vi "Look right.vi"(8 "column":i32, 9 "row":i32, 10 "Tree":T1, 11 "Array":T1[][](array[typedef])) -> (2 "output cluster":T1)   [LabVIEW 2020]
uses:
  tree--cluster.ctl
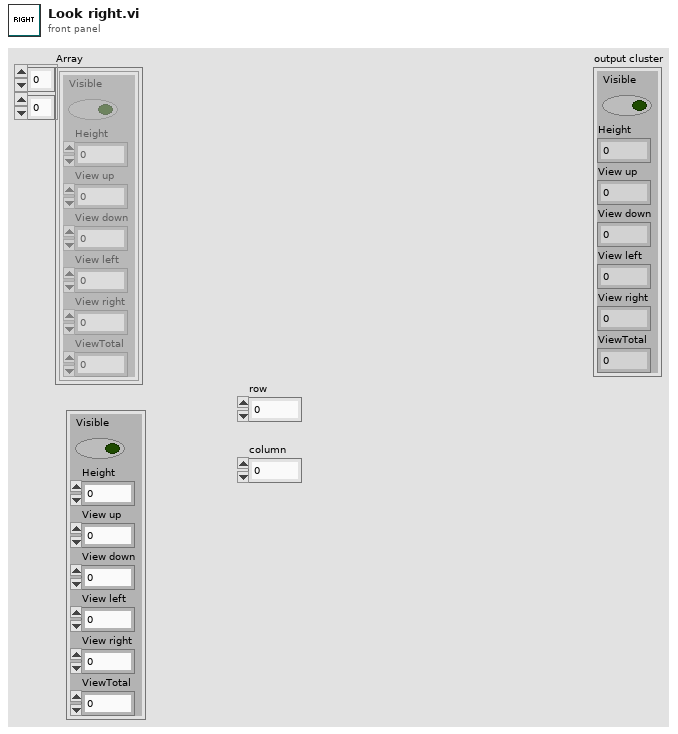
[diagram p1: front panel]
types:
  T1 = typedef "tree--cluster.ctl" = cluster{"Visible":bool, "Height":i32, "View up":i32, "View down":i32, "View left":i32, "View right":i32, "ViewTotal":i32}
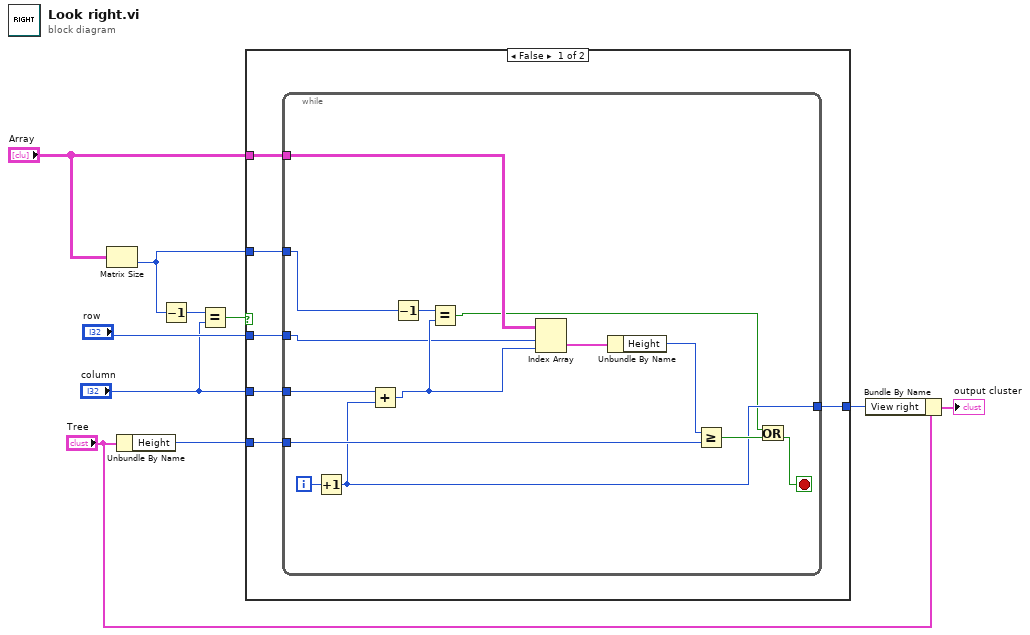
[diagram p0: block diagram]
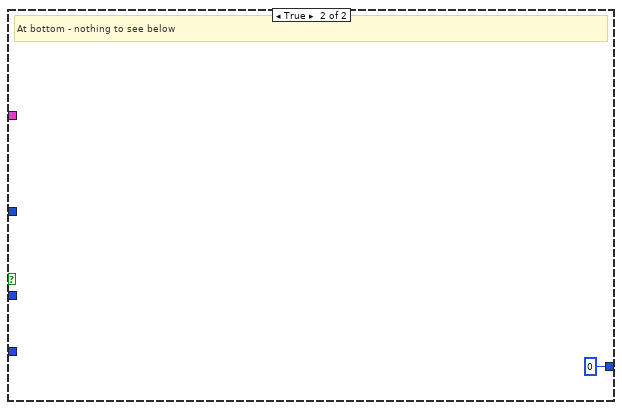
[diagram p2: hidden frame]
diagram:
  n1 = Matrix Size(0:"Array") -> (2:w2:i32)  [unwired: 1 out]
  n2 = Unbundle By Name("Tree") -> ("Height"=w10:i32)
  n3 = Decrement(x=w2) -> (x-1=w5:i32)
  n4 = Equal?(x=w5, y="column") -> (x = y?=w4:bool)
  n5 = case shown="False" w4 {
    tunnel: w10 -> [w16 _]
    tunnel: "column" -> [w15 _]
    tunnel: "row" -> [w14 _]
    tunnel: [w13 0] -> w8
    tunnel: "Array" -> [w12 _]
    tunnel: w2 -> [w11 _]
    frame False {
      n6 = while {
        tunnel: w16 -> [w26]
        tunnel: w12 -> [w30]
        tunnel: w15 -> [w19]
        tunnel: w14 -> [w17]
        tunnel: [w24] -> w13
        tunnel: w11 -> [w22]
        i -> [w29]
        stop <- w21 stop-if-true
        n7 = Increment(x=w29) -> (x+1=w24:i32)
        n8 = Add(x=w19, y=w24) -> (x+y=w18:i32)
        n9 = Decrement(x=w22) -> (x-1=w23:i32)
        n10 = Equal?(x=w23, y=w18) -> (x = y?=w20:bool)
        n11 = Index Array(array=w30, index (row)=w17, index (col)=w18) -> (element=w28:T1)
        n12 = Unbundle By Name(w28) -> ("Height"=w27:i32)
        n13 = Greater Or Equal?(x=w27, y=w26) -> (x >= y?=w25:bool)
        n14 = Or(x=w20, y=w25) -> (x .or. y?=w21:bool)
      }
    }
    frame True {
      # "At bottom - nothing to see below"
    }
  }
  n15 = Bundle By Name(cluster="Tree", "View right"=w8) -> (→"output cluster":T1)
